vi "apply key value pairs.vi"(8 "error in":errorcluster, 9 "values":string[](array[string]), 10 "keys":string[](array[string]), 11 "Watchdog runtime in":refnum<class "Watchdog runtime.lvclass">) -> (0 "error out":errorcluster, 3 "Watchdog runtime out":refnum<class "Watchdog runtime.lvclass">)   [LabVIEW 2013, in "Watchdog runtime.lvclass"]
uses:
  Watchdog runtime.lvclass
  Watchdog runtime.lvclass/Watchdog runtime.ctl
  <vilib>/NI/Configuration Framework/NISE_CEF_TreeControl.lvlib
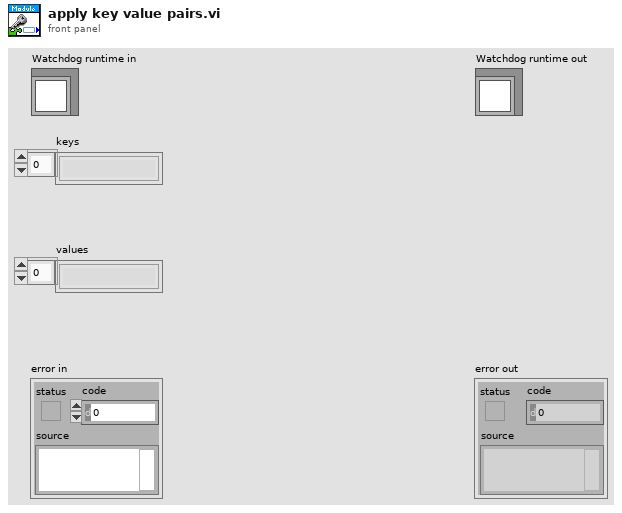
[diagram p1: front panel]
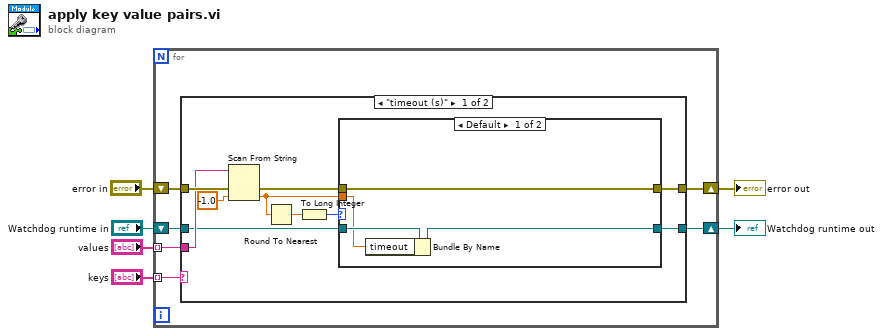
[diagram p0: block diagram]
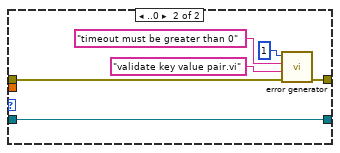
[diagram p2: hidden frame]
diagram:
  n1 = for {
    shift-right: [w10] -> w4
    shift-left: "Watchdog runtime in" -> [w11]
    shift-right: [w9] -> w3
    shift-left: "error in" -> [w12]
    tunnel: "values" -> [w8] mode=indexing
    tunnel: "keys" -> [w7] mode=indexing
    n2 = case shown="\"timeout (s)\"" w7 {
      tunnel: [w22 w34] -> w9
      tunnel: [w14 w33] -> w10
      tunnel: w12 -> [w21 w34]
      tunnel: w8 -> [w19 _]
      tunnel: w11 -> [w15 w33]
      frame "timeout (s)" {
        n3 = Scan From String(input string=w19, error in=w21, default 1=-1.0 ("default value 1")) -> (error out=w20:errorcluster, output 1=w13:dbl)  [unwired: 2 in, 2 out]
        n4 = Round To Nearest(number=w13) -> (nearest integer value=w17:dbl)
        n5 = To Long Integer(number=w17) -> (32bit integer=w16:i32)
        n6 = case shown="Default" w16 {
          tunnel: [w26 w31] -> w22
          tunnel: w20 -> [w26 w29]
          tunnel: w15 -> [w25 w27]
          tunnel: [w24 w27] -> w14
          tunnel: w13 -> [w23 _]
          frame Default {
            n7 = Bundle By Name(cluster=w25, "timeout"=w23) -> (w24:refnum<class "Watchdog runtime.lvclass">)
          }
          frame ..0 {
            n8 = call <vilib>:"error generator.vi"("error in"=w29, "source"="validate key value pair.vi", "append error message"="timeout must be greater than 0", "error code (0)"=1) -> ("error out"=w31:errorcluster)  [unwired: 5 in]
          }
        }
      }
      frame Default {
      }
    }
  }
  "error out" <- w3
  "Watchdog runtime out" <- w4
